vi "Previous Station Check.vi"() -> ()   [LabVIEW 2015]
uses:
  Utility/RPT.ctl
  <vilib>/Utility/error.llb/whitespace.ctl
  <vilib>/addons/database/Connection.llb/DB Tools Open Connec (String).vi
  Galobal variable_TI.vi
  <vilib>/Utility/file.llb/Read Delimited Spreadsheet (string).vi
  Project Setup/Globle Variable/GR_Servo.vi
  <vilib>/Utility/file.llb/Write Delimited Spreadsheet (string).vi
  <vilib>/addons/database/NI_Database_API.lvlib
panel:
  out "error out 5":errorcluster
  out "Data Read":string[][](array[string])
  out "error out 4":errorcluster
  out "size(s)":i32
  out "error out 3":errorcluster
  out "error out":errorcluster
  in  "stop":bool
  in  "RPT":T1
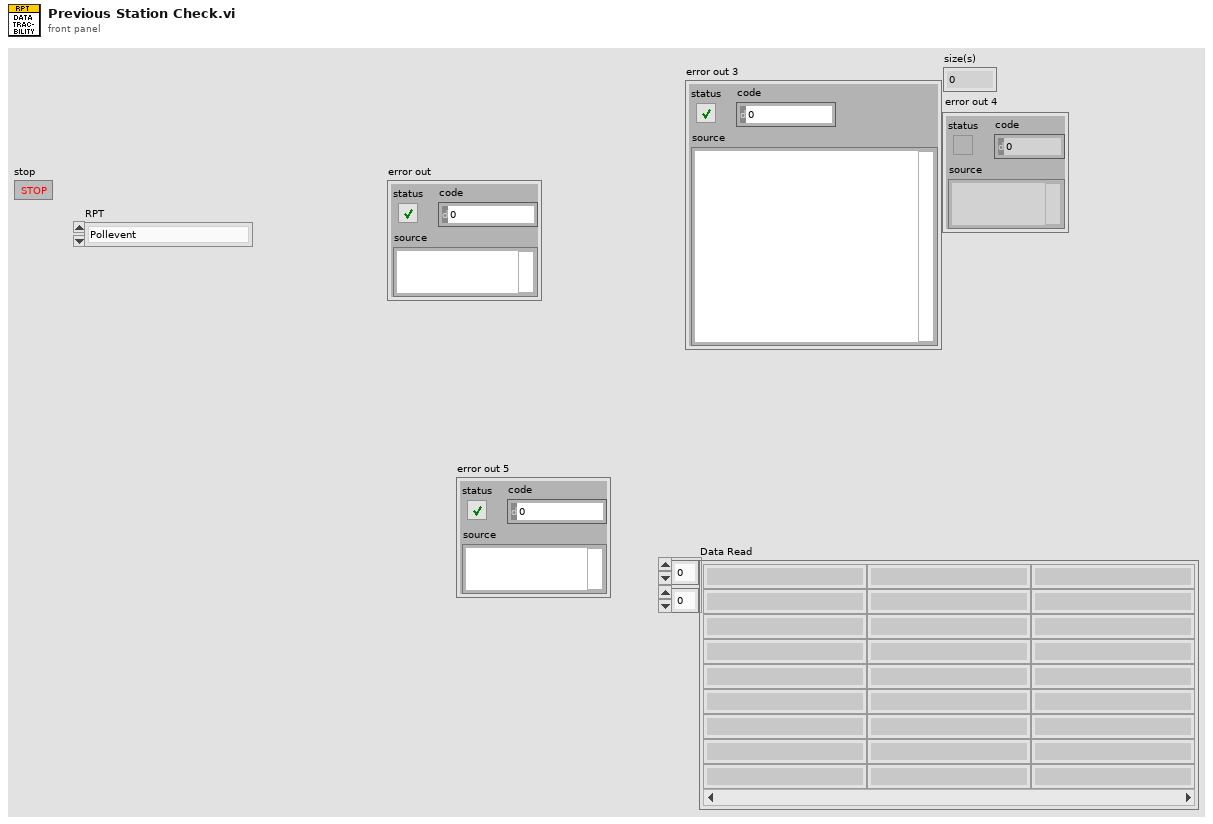
[diagram p1: front panel]
types:
  T1 = typedef "RPT.ctl" = enum16{"Pollevent", "Read", "Write", "Delete"}
  T2 = cluster{"Stn Name":string, "date":string, "time":string, "Operator id":string, "Shift":string, "Error Code":string, "Fail count":string, "Rework":string, "NA":string, "Tested":string}
  T3 = typedef "NI_Database_API.lvlib/Conn ObjectReference.ctl" = refnum<k1>
  T4 = enum16{"open", "replace", "create", "open or create", "replace or create", "replace or create with confirmation"}
  T5 = typedef "whitespace.ctl" = u16
  T6 = cluster{"[0]":void, "[1]":void, "[2]":void, "[3]":void, "[4]":void, "[5]":void, "[6]":void, "[7]":void, "[8]":void, "[9]":void, "[10]":void, "[11]":void, "[12]":void, "[13]":void, "[14]":void, "[15]":void}
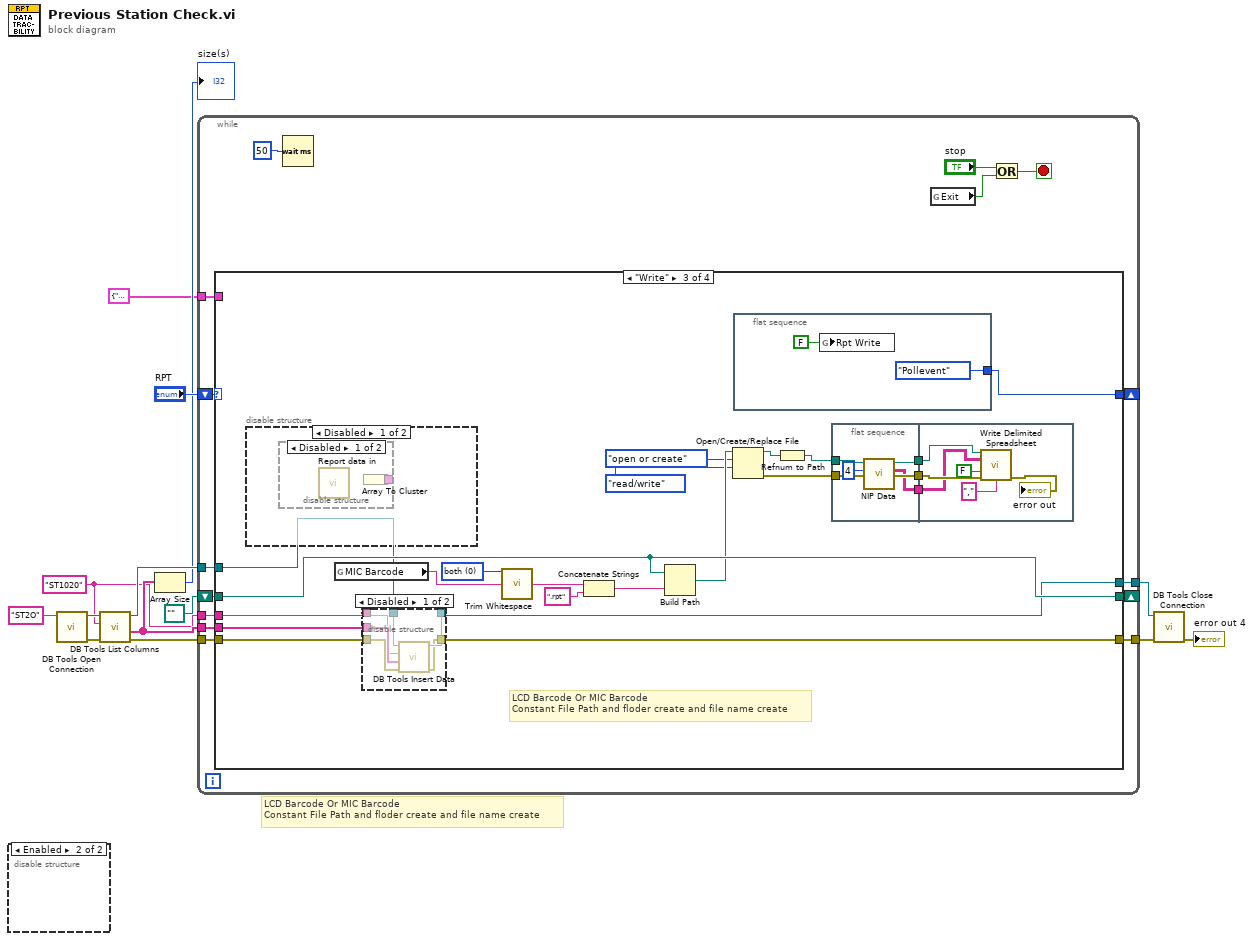
[diagram p0: block diagram]
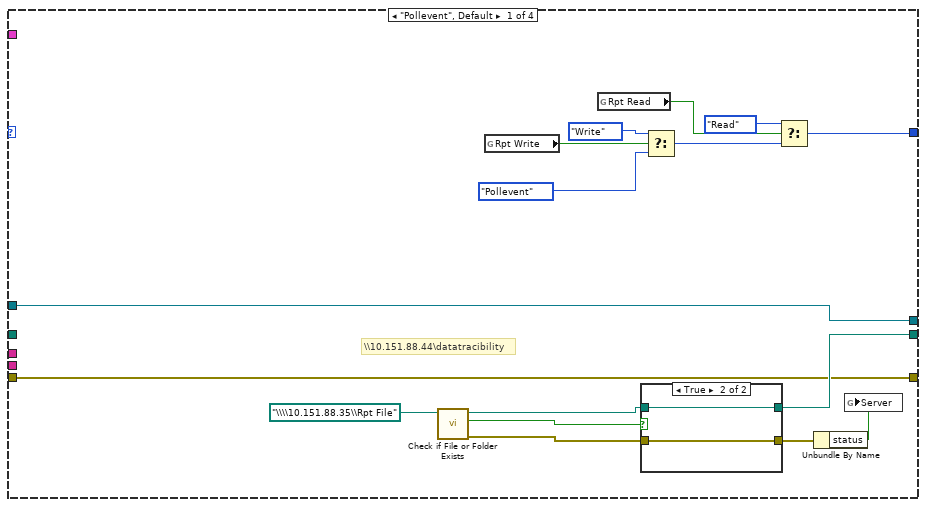
[diagram p2: hidden frame]
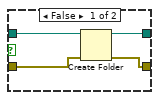
[diagram p3: hidden frame]
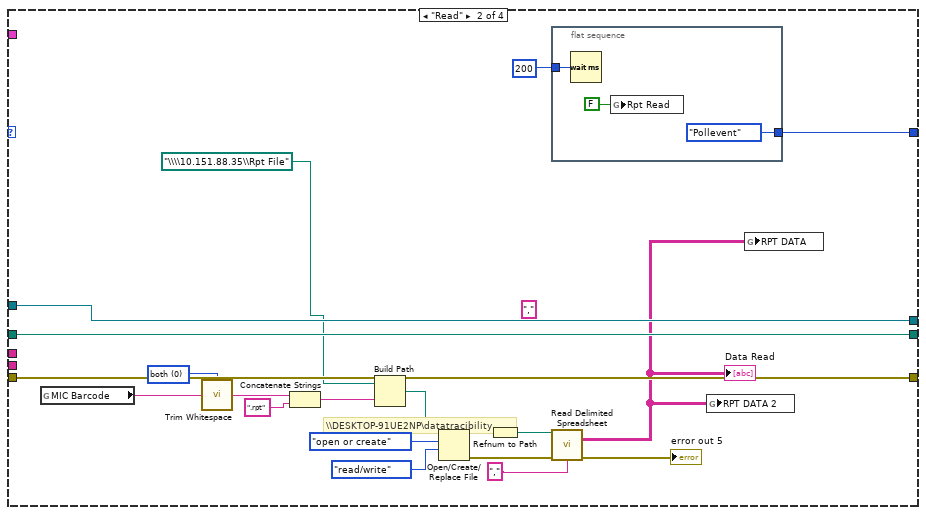
[diagram p4: hidden frame]
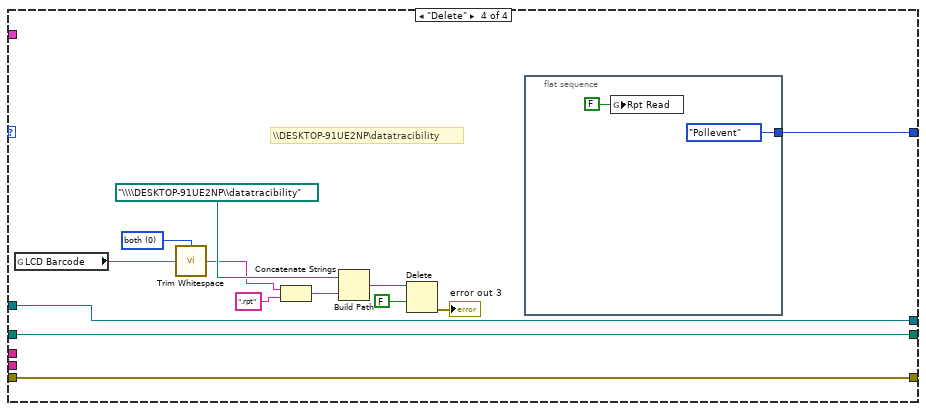
[diagram p8: hidden frame]
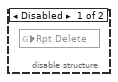
[diagram p9: hidden frame]
diagram:
  w6 = "ST1020" ("table")
  # "LCD Barcode Or MIC Barcode \nConstant File Path and floder create and file name create"
  n1 = disable-structure shown="Enabled" {
    frame Disabled {
      n2 = global read "Galobal variable_TI.vi" "Rpt Delete"() -> ()  [unwired: 1 in]
    }
    frame Enabled {
    }
  }
  n3 = call-poly <vilib>:"DB Tools Open Connection.vi"("connection information"="ST2O" ("string")) -> ("error out"=w11:errorcluster, "connection reference"=w12:T3)  [unwired: 7 in]
  n4 = call <vilib>:"DB Tools List Columns.vi"("error in (no error)"=w11, "table"=w6, "connection reference"=w12) -> ("error out"=w8:errorcluster, "columns"=w7:string[], "connection reference out"=w9:T3)  [unwired: 1 in, 1 out]
  n5 = Array Size(array=w7) -> (size(s)=→"size(s)":i32)
  n6 = while {
    shift-right: [w29] -> _
    shift-left: "RPT" -> [w28]
    shift-right: [w27] -> _
    shift-left: path "" ("created path") -> [w26]
    tunnel: w9 -> [w21]
    tunnel: w8 -> [w20]
    tunnel: w7 -> [w19]
    tunnel: w6 -> [w18]
    tunnel: [w17] -> w5
    tunnel: [w16] -> w4
    tunnel: T2 {"Stn Name"="", "date"="", "time"="", "Operator id"="", "Shift"="", "Error Code"="", "Fail count"="", "Rework"="", "NA"="", "Tested"=""} ("Write Data") -> [w15]
    stop <- w22 stop-if-true
    n7 = case shown="\"Write\"" w28 {
      tunnel: [w39 w71 w96 w129] -> w29
      tunnel: [w34 w70 w93 w126] -> w27
      tunnel: w26 -> [_ w70 w93 w126]
      tunnel: w21 -> [w33 w68 w87 w122]
      tunnel: w20 -> [w32 w67 w86 w121]
      tunnel: w19 -> [_ _ w85 _]
      tunnel: w18 -> [_ _ w84 _]
      tunnel: [w33 w68 w83 w122] -> w17
      tunnel: [w32 w67 w82 w121] -> w16
      tunnel: w15 -> [_ _ _ _]
      frame "Pollevent", Default {
        # "\\\\10.151.88.44\\datatracibility"
        n8 = call <vilib>:"Check if File or Folder Exists.vi"("path"=path "\\\\10.151.88.35\\Rpt File" ("base path")) -> ("error out"=w35:errorcluster, "file or folder exists?"=w37:bool, "dup path"=w36:path)  [unwired: 8 in]
        n9 = global read "Galobal variable_TI.vi" "Rpt Write"() -> (w43:bool)
        n10 = global read "Galobal variable_TI.vi" "Rpt Read"() -> (w44:bool)
        n11 = case shown="True" w37 {
          tunnel: w36 -> [w49 w51]
          tunnel: w35 -> [w48 w50]
          tunnel: [w47 w51] -> w34
          tunnel: [w46 w50] -> w31
          frame False {
            n12 = Create Folder(path (use dialog)=w49, error in=w48) -> (created path=w47:path, error out=w46:errorcluster)  [unwired: 1 in, 1 out]
          }
          frame True {
          }
        }
        n13 = Select(t=RPT."Write" ("RPT"), s=w43, f=RPT."Pollevent" ("RPT")) -> (s? t:f=w41:T1)
        n14 = Select(t=RPT."Read" ("RPT"), s=w44, f=w41) -> (s? t:f=w39:T1)
        n15 = Unbundle By Name(w31) -> ("status"=w30:bool)
        n16 = global write "Galobal variable_TI.vi" "Server"(w30) -> ()
      }
      frame "Read" {
        w61 = T5 0 items=["both", "start of string", "end of string"] ("location (both)")
        (unwired) "," ("delimiter (\\t)")
        # "\\\\DESKTOP-91UE2NP\\datatracibility"
        n17 = global read "Galobal variable_TI.vi" "MIC Barcode"() -> (w60:string)
        n18 = call <vilib>:"Trim Whitespace.vi"("string"=w60, "location (both)"=w61) -> ("trimmed string"=w62:string)
        n19 = Concatenate Strings(w62, ".rpt" ("string")) -> (w55:string)
        n20 = Build Path(base path=path "\\\\10.151.88.35\\Rpt File", name or relative path=w55) -> (appended path=w56:path)
        n21 = Open/Create/Replace File(file path (use dialog)=w56, operation (0:open)=T4."open or create", access (0:read/write)=enum16{"read/write", "read-only", "write-only"}."read/write") -> (refnum out=w63:refnum<file>, error out=w59:errorcluster)  [unwired: 3 in, 1 out]
        n22 = Refnum to Path(1:w63) -> (0:w64:path)
        n23 = flat-sequence {
          tunnel: [RPT."Pollevent" ("RPT")] -> w71
          tunnel: u32 200 ("milliseconds to wait") -> [w72]
          frame #0 {
            n24 = Wait (ms)(milliseconds to wait=w72) -> ()  [unwired: 1 out]
            n25 = global write "Galobal variable_TI.vi" "Rpt Read"(FALSE ("Rpt Read")) -> ()
          }
        }
        n26 = call-poly <vilib>:"Read Delimited Spreadsheet.vi"("file path (dialog if empty)"=w64, "error in (no error)"=w59, "delimiter (\\t)"="," ("delimiter (\\t)")) -> ("all rows"=w52:string[][], "error out"=→"error out 5":errorcluster)  [unwired: 7 in, 4 out]
        "Data Read" <- w52
        n27 = global write "GR_Servo.vi" "RPT DATA 2"(w52) -> ()
        n28 = global write "GR_Servo.vi" "RPT DATA"(w52) -> ()
      }
      frame "Write" {
        w79 = T5 0 items=["both", "start of string", "end of string"] ("location (both)")
        # "LCD Barcode Or MIC Barcode \nConstant File Path and floder create and file name create"
        n29 = disable-structure shown="Disabled" {
          frame Disabled {
            n30 = disable-structure shown="Disabled" {
              disable-tunnel: [w108 _] -> _
              frame Disabled {
                n31 = call "Report data in.vi"() -> ()  [unwired: 11 in, 1 out]
                n32 = Array To Cluster() -> (cluster=w108:T6)  [unwired: 1 in]
              }
              frame Enabled {
              }
            }
          }
          frame Enabled {
          }
        }
        n33 = global read "Galobal variable_TI.vi" "MIC Barcode"() -> (w81:string)
        n34 = disable-structure shown="Disabled" {
          disable-tunnel: w87 -> [w114 _]
          disable-tunnel: w86 -> [w113 _]
          disable-tunnel: w85 -> [w112 _]
          disable-tunnel: w84 -> [w111 _]
          disable-tunnel: [w110 _] -> w83
          disable-tunnel: [w109 _] -> w82
          frame Disabled {
            n35 = call <vilib>:"DB Tools Insert Data.vi"("error in (no error)"=w113, "columns"=w112, "table"=w111, "connection reference"=w114) -> ("error out"=w109:errorcluster, "connection reference out"=w110:T3)  [unwired: 6 in]
          }
          frame Enabled {
          }
        }
        n36 = call <vilib>:"Trim Whitespace.vi"("string"=w81, "location (both)"=w79) -> ("trimmed string"=w80:string)
        n37 = Concatenate Strings(w80, ".rpt" ("string")) -> (w94:string)
        n38 = Build Path(base path=w93, name or relative path=w94) -> (appended path=w92:path)
        n39 = Open/Create/Replace File(file path (use dialog)=w92, operation (0:open)=T4."open or create", access (0:read/write)=enum16{"read/write", "read-only", "write-only"}."read/write") -> (refnum out=w89:refnum<file>, error out=w88:errorcluster)  [unwired: 3 in, 1 out]
        n40 = flat-sequence {
          tunnel: [RPT."Pollevent" ("RPT")] -> w96
          frame #0 {
            n41 = global write "Galobal variable_TI.vi" "Rpt Write"(FALSE ("Rpt Read")) -> ()
          }
        }
        n42 = Refnum to Path(1:w89) -> (0:w78:path)
        n43 = flat-sequence {
          tunnel: w78 -> [w99]
          tunnel: w88 -> [w101]
          tunnel: [w101] -> w77
          tunnel: [w98] -> w76
          tunnel: [w100] -> w75
          tunnel: w77 -> [w107]
          tunnel: w76 -> [w103]
          tunnel: w75 -> [w102]
          frame #0 {
            n44 = call "NIP Data.vi"("index (row)"=4, "file path (dialog if empty)"=w99) -> ("Data"=w100:string[][], "file path (dialog if empty) 2"=w98:path)  [unwired: 8 in]
          }
          frame #1 {
            n45 = call-poly <vilib>:"Write Delimited Spreadsheet.vi"("file path (dialog if empty)"=w103, "2D data"=w102, "append to file? (F)"=FALSE, "error in (no error)"=w107, "delimiter (\\t)"="," ("delimiter (\\t)")) -> ("error out"=→"error out":errorcluster)  [unwired: 9 in, 1 out]
          }
        }
      }
      frame "Delete" {
        w119 = T5 0 items=["both", "start of string", "end of string"] ("location (both)")
        # "\\\\DESKTOP-91UE2NP\\datatracibility"
        n46 = global read "Galobal variable_TI.vi" "LCD Barcode"() -> (w118:string)
        n47 = call <vilib>:"Trim Whitespace.vi"("string"=w118, "location (both)"=w119) -> ("trimmed string"=w117:string)
        n48 = Concatenate Strings(w117, ".rpt" ("string")) -> (w127:string)
        n49 = Build Path(base path=path "\\\\DESKTOP-91UE2NP\\datatracibility", name or relative path=w127) -> (appended path=w125:path)
        n50 = Delete(path (use dialog)=w125, confirm (F)=FALSE) -> (error out=→"error out 3":errorcluster)  [unwired: 3 in, 2 out]
        n51 = flat-sequence {
          tunnel: [RPT."Pollevent" ("RPT")] -> w129
          frame #0 {
            n52 = global write "Galobal variable_TI.vi" "Rpt Read"(FALSE ("Rpt Read")) -> ()
          }
        }
      }
    }
    n53 = Wait (ms)(milliseconds to wait=u32 50) -> ()  [unwired: 1 out]
    n54 = global read "Galobal variable_TI.vi" "Exit"() -> (w24:bool)
    n55 = Or(x="stop", y=w24) -> (x .or. y?=w22:bool)
  }
  n56 = call <vilib>:"DB Tools Close Connection.vi"("error in (no error)"=w4, "connection reference"=w5) -> ("error out"=→"error out 4":errorcluster)  [unwired: 5 in]
